vi "Unflatten Compiled Data.vi"(8 "error in (no error)":errorcluster, 9 "Compiled.Settings":T6 {"Inline Execution Unit Compiled Information"."Outgoing Data References"."Data Reference" format="%.0x"; "Inline Execution Unit Compiled Information"."Incoming Data References" format="%.0x"}, 10 "RTStateVariables in":T1 {"Inline Execution Units"."Outgoing Data References"."Data Reference" format="%.0x"; "Inline Execution Units"."Incoming Data References" format="%.0x"}, 11 "Item Ref in":T9 format="%.0x") -> (0 "error out":errorcluster, 2 "RTStateVariables out":T1 {"Inline Execution Units"."Outgoing Data References"."Data Reference" format="%.0x"; "Inline Execution Units"."Incoming Data References" format="%.0x"}, 3 "Item Ref out":T9 format="%.0x")   [LabVIEW 2020, in "Communication Bus Template Engine.lvlib"]
uses:
  Communication Bus Template Engine.lvlib
  <vilib>/NI VeriStand/Custom Device API/Custom Device Item Ref.ctl
  RTStateVariables.ctl
  <vilib>/NI/NIVS Inline Async API/_VS Inline Async API/VS Inline Async API/VS Inline Async API.lvclass
  Shared/Compiled.Settings.ctl
  Shared/Inline Execution Unit Compiled Information.ctl
  <vilib>/NI VeriStand/Custom Device API/Custom Device API.lvlib
  <vilib>/NI VeriStand/Custom Device API/Data Reference.ctl
  <vilib>/NI VeriStand/Custom Device API/Block Data Reference.ctl
  Shared/Communication Bus Template Shared.lvlib
  Includes/Communication Bus Interfaces.lvlibp/Interfaces/Execution Unit/Execution Unit/Execution Unit.lvclass
  Inline Execution Unit Runtime Information.ctl
  Shared/Asynchronous Execution Unit Compiled Information.ctl
  Asynchronous Execution Unit Runtime Information.ctl
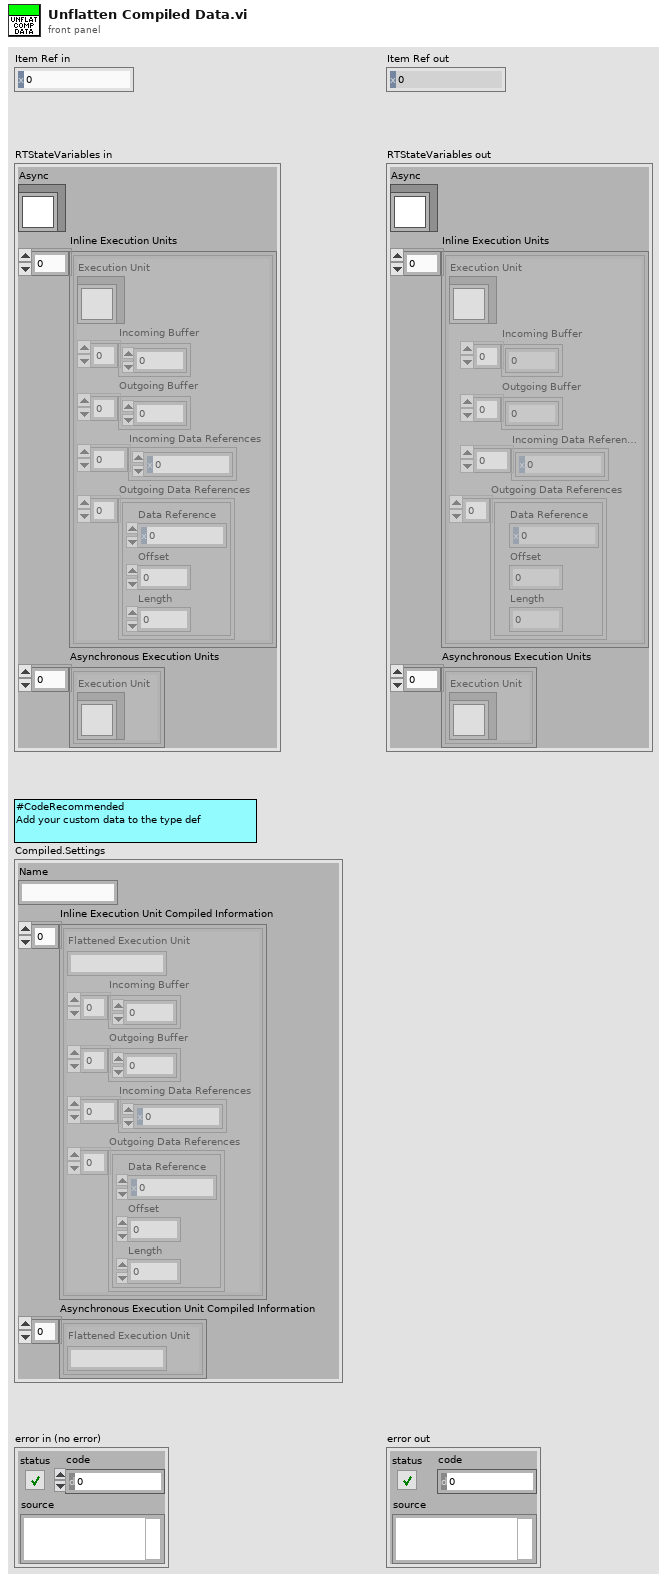
[diagram p1: front panel]
types:
  T1 = typedef "Communication Bus Template Engine.lvlib/RTStateVariables.ctl" = cluster{"Async":refnum<class "VS Inline Async API.lvclass">, "Inline Execution Units":T2[], "Asynchronous Execution Units":T5[]}
  T2 = typedef "Communication Bus Template Engine.lvlib/Inline Execution Unit Runtime Information.ctl" = cluster{"Execution Unit":refnum<class "Execution Unit.lvclass">, "Incoming Buffer":dbl[], "Outgoing Buffer":dbl[], "Incoming Data References":T3[], "Outgoing Data References":T4[]}
  T3 = typedef "Custom Device API.lvlib/Data Reference.ctl" = i32
  T4 = typedef "Custom Device API.lvlib/Block Data Reference.ctl" = cluster{"Data Reference":T3, "Offset":u64, "Length":u64}
  T5 = typedef "Communication Bus Template Engine.lvlib/Asynchronous Execution Unit Runtime Information.ctl" = cluster{"Execution Unit":refnum<class "Execution Unit.lvclass">}
  T6 = typedef "Communication Bus Template Shared.lvlib/Compiled.Settings.ctl" = cluster{"Name":string, "Inline Execution Unit Compiled Information":T7[], "Asynchronous Execution Unit Compiled Information":T8[]}
  T7 = typedef "Communication Bus Template Shared.lvlib/Inline Execution Unit Compiled Information.ctl" = cluster{"Flattened Execution Unit":string, "Incoming Buffer":dbl[], "Outgoing Buffer":dbl[], "Incoming Data References":T3[], "Outgoing Data References":T4[]}
  T8 = typedef "Communication Bus Template Shared.lvlib/Asynchronous Execution Unit Compiled Information.ctl" = cluster{"Flattened Execution Unit":string}
  T9 = typedef "Custom Device API.lvlib/Custom Device Item Ref.ctl" = u64
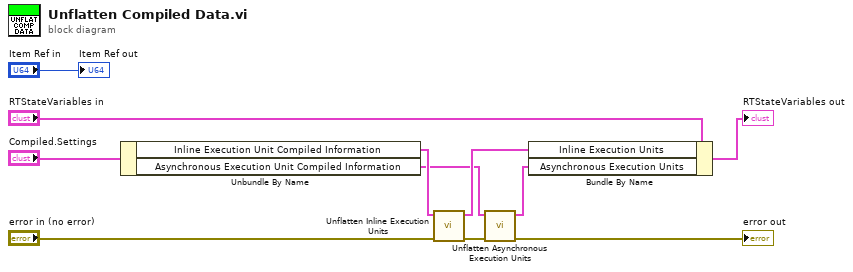
[diagram p0: block diagram]
diagram:
  n1 = Unbundle By Name("Compiled.Settings") -> ("Inline Execution Unit Compiled Information"=w5:T7[], "Asynchronous Execution Unit Compiled Information"=w4:T8[])
  n2 = call "Unflatten Inline Execution Units.vi"("error in (no error)"="error in (no error)", "Compiled Inline Execution Units"=w5) -> ("error out"=w2:errorcluster, "Inline Execution Units"=w6:T2[])  [unwired: 8 in]
  n3 = call "Unflatten Asynchronous Execution Units.vi"("error in (no error)"=w2, "Compiled Asynchronous Execution Units"=w4) -> ("error out"=→"error out":errorcluster, "Asynchronous Execution Units"=w3:T5[])  [unwired: 8 in]
  n4 = Bundle By Name(cluster="RTStateVariables in", "Inline Execution Units"=w6, "Asynchronous Execution Units"=w3) -> (→"RTStateVariables out":T1)
  "Item Ref out" <- "Item Ref in"
